vi "Mark Keys Changed.vi"(10 "Changed keys":string[](array[string]), 11 "ConfigManager.Text in":refnum<class "ConfigManager.Text.lvclass">) -> (3 "ConfigManager.Text out":refnum<class "ConfigManager.Text.lvclass">)   [LabVIEW 2013, in "CfgManager.Text.lvlib" / "ConfigManager.Text.lvclass"]
uses:
  ConfigManager.Text.lvclass
  ConfigManager.Text.lvclass/ConfigManager.Text.ctl
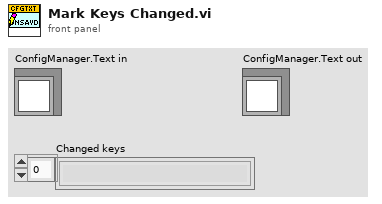
[diagram p1: front panel]
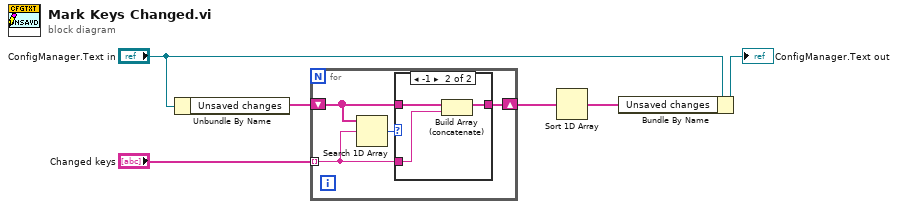
[diagram p0: block diagram]
diagram:
  n1 = Unbundle By Name("ConfigManager.Text in") -> ("Unsaved changes"=w3:string[])
  n2 = for {
    tunnel: "Changed keys" -> [w9] mode=indexing
    shift-right: [w8] -> w2
    shift-left: w3 -> [w10]
    n3 = Search 1D Array(1D array=w10, element=w9) -> (index of element=w7:i32)  [unwired: 1 in]
    n4 = case shown="-1" w7 {
      tunnel: w10 -> [w11 w14]
      tunnel: w9 -> [_ w13]
      tunnel: [w11 w12] -> w8
      frame Default {
      }
      frame -1 {
        n5 = Build Array (concatenate)(w14, w13) -> (w12:string[])
      }
    }
  }
  n6 = Sort 1D Array(array=w2) -> (sorted array=w1:string[])
  n7 = Bundle By Name(cluster="ConfigManager.Text in", "Unsaved changes"=w1) -> (→"ConfigManager.Text out":refnum<class "ConfigManager.Text.lvclass">)
